vi "Basic Accuracy Parameter.vi"(8 "error in (no error)":errorcluster, 10 "Impedance Z (10m)":dbl=0.01 min=0.01 max=100000000.0 format="%^.2e", 11 "VISA resource name":refnum<visa-resource-name>) -> (0 "error out":errorcluster, 2 "Parameter A":dbl format="%.3f", 3 "VISA resource name out":refnum<visa-resource-name>, 5 "Frequency Used":dbl format="%.2f")   [LabVIEW 2015, in "Agilent 428X Series.lvlib"]
doc: "This VI is to calculate the value of parameter A for accuracy measurement,\n\nDisclaimer: All accuracy calculation VI's are not part of the original \n driver. They are provided for supplementry purpose only.\n If user desires very high accuracy data, please do or \n check the calculation seperately."
uses:
  Agilent 428X Series.lvlib
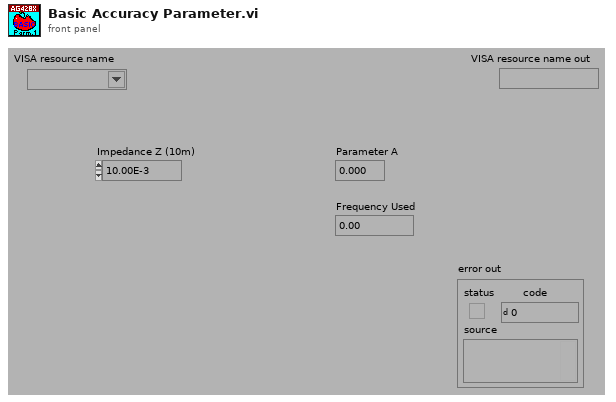
[diagram p1: front panel]
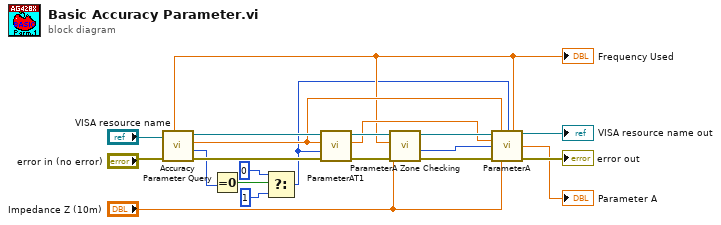
[diagram p0: block diagram]
diagram:
  n1 = call "Accuracy Parameter Query.vi"("error in (no error)"="error in (no error)", "VISA resource name"="VISA resource name") -> ("error out"=w18:errorcluster, "Time Integration"=w5:u8, "Voltage Level"=w8:dbl, "VISA resource name out"=w19:refnum<visa-resource-name>, "Frequency"=w7:dbl)  [unwired: 4 in, 1 out]
  "Frequency Used" <- w7
  n2 = Equal To 0?(x=w5) -> (x = 0?=w4:bool)
  n3 = Select(t=i8 0, s=w4, f=i8 1) -> (s? t:f=w1:i8)
  n4 = call "ParameterAT1.vi"("error in (no error)"=w18, "Integ Time (0: Short)"=w1, "Voltage Level (1.0)"=w8, "VISA resource name"=w19) -> ("error out"=w16:errorcluster, "Parameter At1"=w12:dbl, "VISA resource name out"=w17:refnum<visa-resource-name>)  [unwired: 5 in]
  n5 = call "ParameterA Zone Checking.vi"("error in (no error)"=w16, "Impedance Z (10m)"="Impedance Z (10m)", "Frequency (20)"=w7, "VISA resource name"=w17) -> ("error out"=w14:errorcluster, "Zone"=w13:i8, "VISA resource name out"=w15:refnum<visa-resource-name>)  [unwired: 5 in]
  n6 = call "ParameterA.vi"("VISA resource name"=w15, "Voltage Level (1.0)"=w8, "Integ Time (0: Short)"=w1, "Frequency (20)"=w7, "AT1"=w12, "Zone (0)"=w13, "error in (no error)"=w14, "Impedance Z (10m)"="Impedance Z (10m)") -> ("VISA resource name out"=→"VISA resource name out":refnum<visa-resource-name>, "Parameter A"=→"Parameter A":dbl, "error out"=→"error out":errorcluster)  [unwired: 5 in]
